vi "kvCanGet8ByteChannelData.vi"(2 "error in (no error)":errorcluster, 3 "Data Item":T1(ring), 4 "Channel Number":i32) -> (0 "error out":errorcluster, 1 "Data":u8[](array[numeric]) format="%.0x")   [LabVIEW 2022 SP3]
doc: "This VI gets various 8-byte channel data values:\n\nItem \"Card UPC Number\": the UPC (EAN) number for the card. If there is no UPC number, the buffer is filled with zeros. The UPC (EAN) number is coded as a BCD string with the LSB first, so e.g. 733-0130-00122-0 is coded as 0x30001220 0x00073301. \n\nItem \"Transceiver UPC Number\": the UPC (EAN) number for the transceiver. If there is no UPC number, the buffer is filled with zeros. The UPC (EAN) number is coded as a BCD string with the LSB first, so e.g. 733-0130-00122-0 is coded as 0x30001220 0x00073301. \n\nItem \"Card Serial Number\": the serial number of the card. If the card doesn't have a serial number, 0 is returned.\n\nItem \"Transceiver Serial Number\": the serial number of the transceivcer. If the transceivcer doesn't have a serial number, 0 is returned. \n\nItem \"Card Firmware Rev\": the firmware revision number on the card. This number consists of four 16-bit words: the major revision, the minor revision, the release number and the build number, listed in order from the most significant to the least significant. \n\nItem \"Card Hardware Rev\": the hardware revision number on the card. This number consists of four 16-bit words: the major revision, the minor revision, the release number and the build number, listed in order from the most significant to the least significant."
uses:
  canlib32.dll
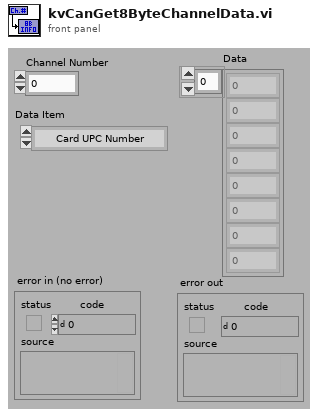
[diagram p1: front panel]
types:
  T1 = enum16{"Card UPC Number", "Card Serial Number", "Transceiver UPC", "Transceiver Serial Number", "Card Firmware Rev", "Card Hardware Rev"}
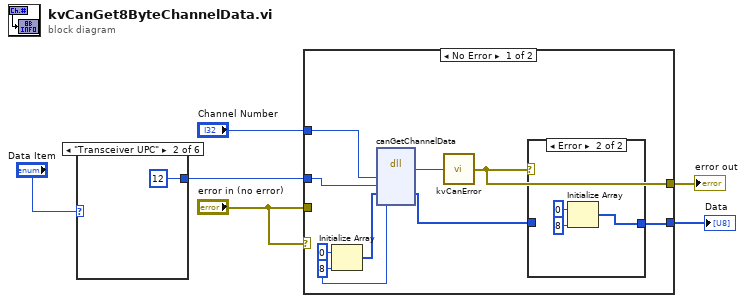
[diagram p0: block diagram]
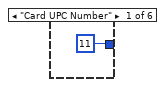
[diagram p2: hidden frame]
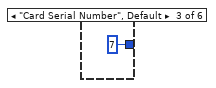
[diagram p3: hidden frame]
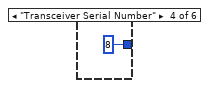
[diagram p4: hidden frame]
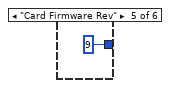
[diagram p5: hidden frame]
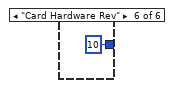
[diagram p6: hidden frame]
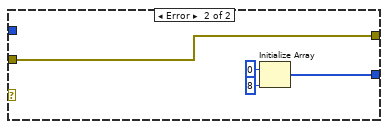
[diagram p8: hidden frame]
diagram:
  n1 = case shown="\"Transceiver UPC\"" "Data Item" {
    tunnel: [11 12 7 8 9 10] -> w1
    frame "Card UPC Number" {
    }
    frame "Transceiver UPC" {
    }
    frame "Card Serial Number", Default {
    }
    frame "Transceiver Serial Number" {
    }
    frame "Card Firmware Rev" {
    }
    frame "Card Hardware Rev" {
    }
  }
  n2 = case shown="No Error" "error in (no error)" {
    tunnel: "error in (no error)" -> [_ w29]
    tunnel: [w19 w29] -> w5
    tunnel: [w18 w26] -> w3
    tunnel: "Channel Number" -> [w21 _]
    tunnel: w1 -> [w13 _]
    frame No Error {
      w16 = 8
      n3 = Initialize Array(u8 0, w16) -> (w14:u8[])
      n4 = dll-call lib="canlib32.dll" fn="canGetChannelData" label="Call canGetChannelData"("channel"=w21, "item"=w13, "buffer"=w14, "bufsize"=w16) -> (w20:i32, "buffer"=w17:u8[])  [unwired: 6 in, 2 out]
      n5 = call "kvCanError.vi"("error code"=w20) -> ("error out"=w19:errorcluster)
      n6 = case shown="Error" w19 {
        tunnel: [w22 w23] -> w18
        tunnel: w17 -> [w22 _]
        frame No Error {
        }
        frame Error {
          n7 = Initialize Array(u8 0, 8) -> (w23:u8[])
        }
      }
    }
    frame Error {
      n8 = Initialize Array(u8 0, 8) -> (w26:u8[])
    }
  }
  "error out" <- w5
  "Data" <- w3
